vi "generate_new_stimulus_array_check.vi"(0 "output cluster":T1, 1 "Input Values cluster":T2) -> (2 "output cluster 2":T1, 3 "Output Values Cluster":T2, 4 "Need new stimulus array?":bool)   [LabVIEW 2015]
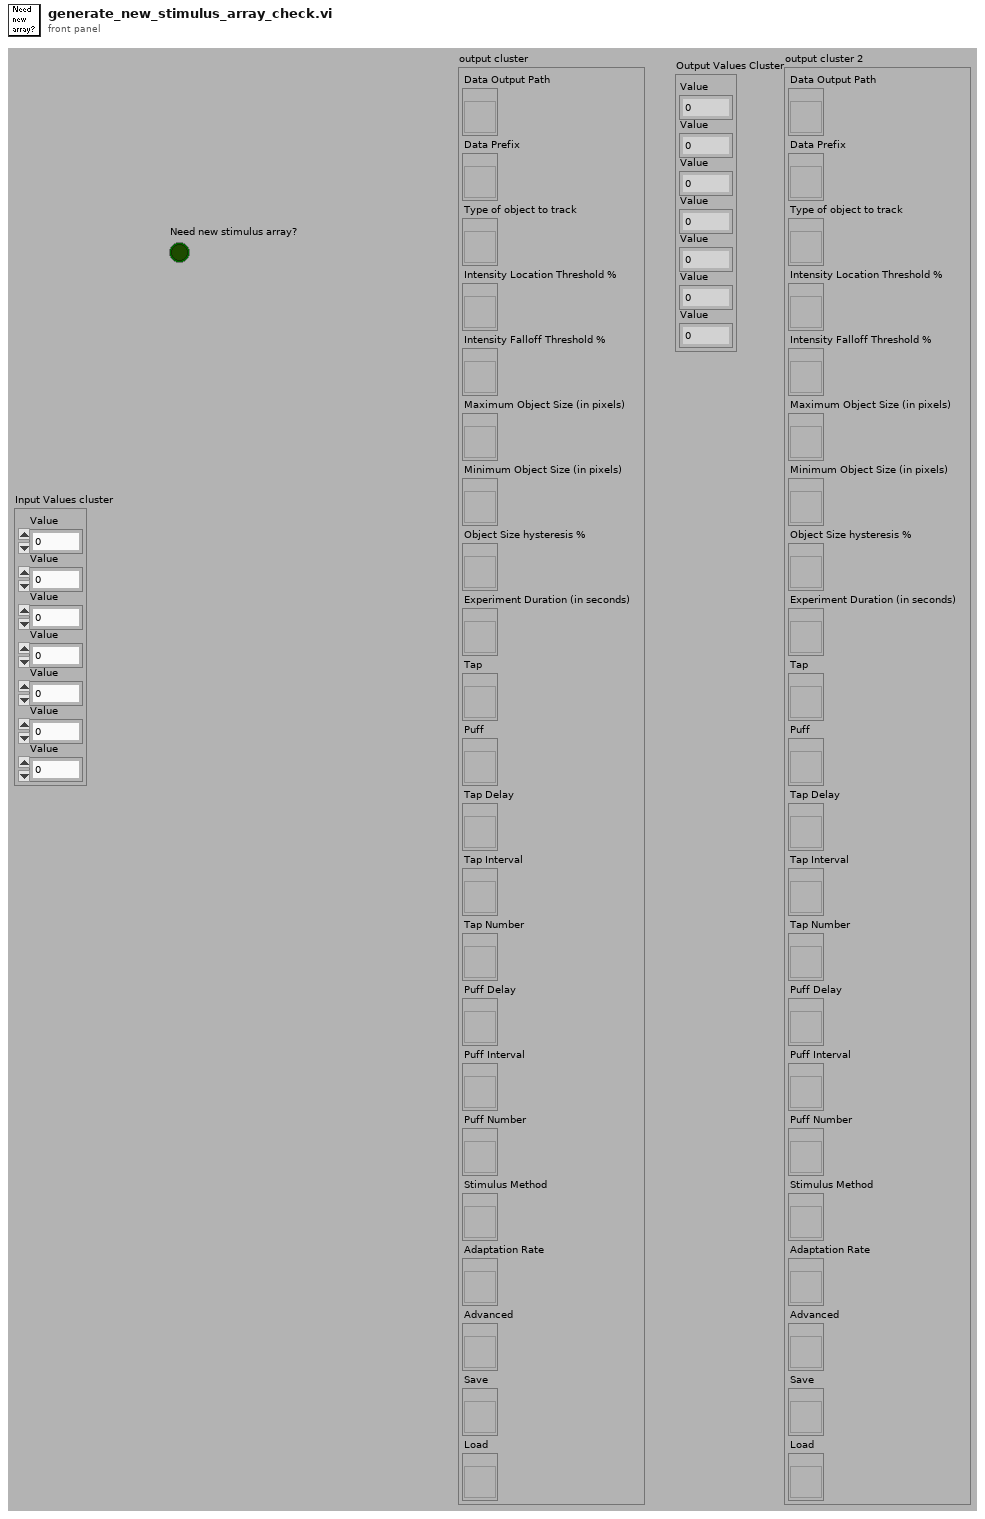
[diagram p1: front panel]
types:
  T1 = cluster{"Data Output Path":refnum<vi>, "Data Prefix":refnum<vi>, "Type of object to track":refnum<vi>, "Intensity Location Threshold %":refnum<vi>, "Intensity Falloff Threshold %":refnum<vi>, "Maximum Object Size (in pixels)":refnum<vi>, "Minimum Object Size (in pixels)":refnum<vi>, "Object Size hysteresis %":refnum<vi>, "Experiment Duration (in seconds)":refnum<vi>, "Tap":refnum<vi>, "Puff":refnum<vi>, "Tap Delay":refnum<vi>, "Tap Interval":refnum<vi>, "Tap Number":refnum<vi>, "Puff Delay":refnum<vi>, "Puff Interval":refnum<vi>, "Puff Number":refnum<vi>, "Stimulus Method":refnum<vi>, "Adaptation Rate":refnum<vi>, "Advanced":refnum<vi>, "Save":refnum<vi>, "Load":refnum<vi>}
  T2 = cluster{"Value":dbl, "Value":dbl, "Value":dbl, "Value":dbl, "Value":dbl, "Value":dbl, "Value":u16}
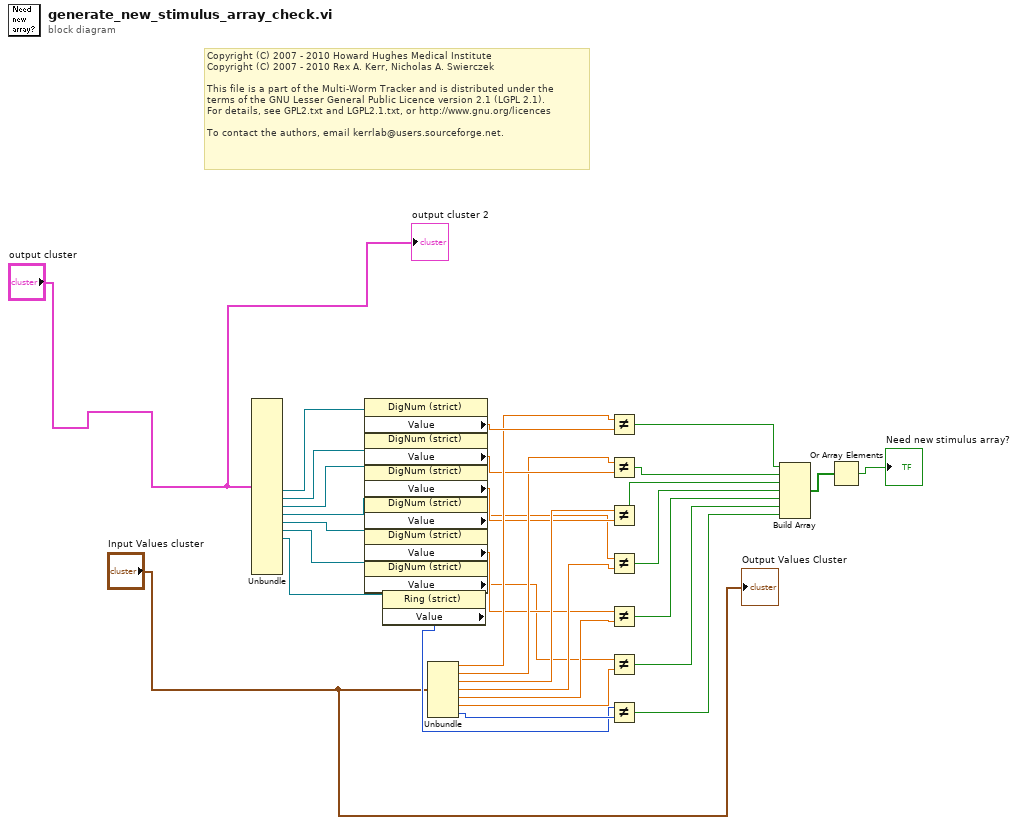
[diagram p0: block diagram]
diagram:
  # "Copyright (C) 2007 - 2010 Howard Hughes Medical Institute\nCopyright (C) 2007 - 2010 Rex A. Kerr, Nicholas A. Swierczek\n \nThis file is a part of the Multi-Worm Tracker and is distributed under the\nterms of the GNU Lesser General Public Licence version 2.1 (LGPL 2.1).\nFor details, see GPL2.txt and LGPL2.1.txt, or http://www.gnu.org/licences\n \nTo contact the authors, email kerrlab@users.sourceforge.net."
  n1 = Unbundle("output cluster") -> ("Tap Delay"=w32:refnum<vi>, "Tap Interval"=w31:refnum<vi>, "Tap Number"=w30:refnum<vi>, "Puff Delay"=w29:refnum<vi>, "Puff Interval"=w28:refnum<vi>, "Puff Number"=w27:refnum<vi>, "Stimulus Method"=w26:refnum<vi>)  [unwired: 15 out]
  n2 = property class="DigNum (strict)"(reference=w32) -> ("Value"=w24:dbl)  [unwired: 1 in, 2 out]
  n3 = property class="DigNum (strict)"(reference=w31) -> ("Value"=w22:dbl)  [unwired: 1 in, 2 out]
  n4 = property class="DigNum (strict)"(reference=w30) -> ("Value"=w19:dbl)  [unwired: 1 in, 2 out]
  n5 = property class="DigNum (strict)"(reference=w29) -> ("Value"=w17:dbl)  [unwired: 1 in, 2 out]
  n6 = property class="DigNum (strict)"(reference=w28) -> ("Value"=w15:dbl)  [unwired: 1 in, 2 out]
  n7 = property class="DigNum (strict)"(reference=w27) -> ("Value"=w13:dbl)  [unwired: 1 in, 2 out]
  n8 = property class="Ring (strict)"(reference=w26) -> ("Value"=w11:u16)  [unwired: 1 in, 2 out]
  n9 = Unbundle("Input Values cluster") -> ("Value"=w23:dbl, "Value"=w21:dbl, "Value"=w20:dbl, "Value"=w16:dbl, "Value"=w18:dbl, "Value"=w14:dbl, "Value"=w12:u16)
  n10 = Not Equal?(x=w23, y=w24) -> (x != y?=w7:bool)
  n11 = Not Equal?(x=w21, y=w22) -> (x != y?=w10:bool)
  n12 = Not Equal?(x=w20, y=w19) -> (x != y?=w6:bool)
  n13 = Not Equal?(x=w17, y=w16) -> (x != y?=w5:bool)
  n14 = Not Equal?(x=w15, y=w18) -> (x != y?=w4:bool)
  n15 = Not Equal?(x=w13, y=w14) -> (x != y?=w3:bool)
  n16 = Not Equal?(x=w11, y=w12) -> (x != y?=w2:bool)
  n17 = Build Array(w7, w10, w6, w5, w4, w3, w2) -> (w9:bool[])
  n18 = Or Array Elements(Boolean array=w9) -> (logical OR=→"Need new stimulus array?":bool)
  "Output Values Cluster" <- "Input Values cluster"
  "output cluster 2" <- "output cluster"
